vi "Obtain Thread.vi"(8 "error in (no error)":errorcluster, 9 "timeout in ms (0)":i32 format="%d ms", 11 "Thread Pool in":refnum<class "Thread Pool.lvclass">) -> (0 "error out":errorcluster, 1 "timed out?":bool, 2 "Thread":refnum<class "Thread.lvclass">, 3 "Thread Pool out":refnum<class "Thread Pool.lvclass">)   [LabVIEW 2017, in "DSF Core.lvlib" / "Thread Pool.lvclass"]
uses:
  Thread Pool.lvclass
  Thread/Thread.lvclass
  Thread Pool.lvclass/Thread Pool.ctl
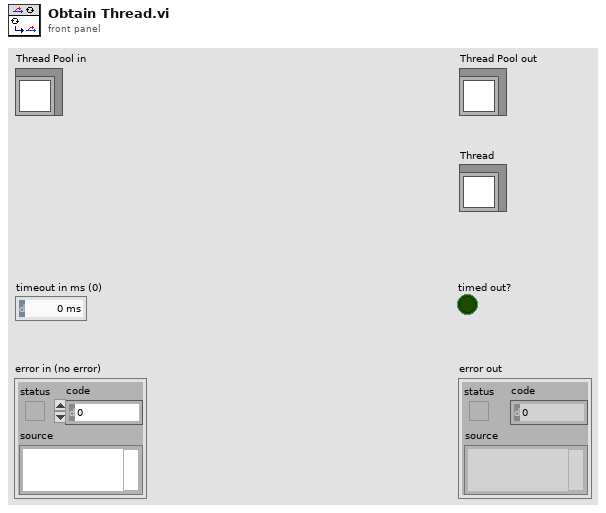
[diagram p1: front panel]
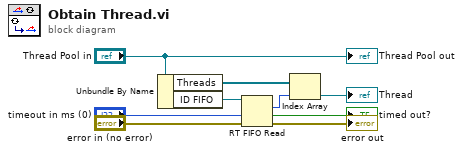
[diagram p0: block diagram]
diagram:
  n1 = Unbundle By Name("Thread Pool in") -> ("Threads"=w5:refnum<class "Thread.lvclass">[], "ID FIFO"=w8:refnum<k33>)
  n2 = RT FIFO Read(0:w8, 2:"timeout in ms (0)", 3:"error in (no error)") -> (9:w4:i32, 10:→"timed out?":bool, 11:→"error out":errorcluster)  [unwired: 1 in, 2 out]
  n3 = Index Array(array=w5, index=w4) -> (element=→"Thread":refnum<class "Thread.lvclass">)
  "Thread Pool out" <- "Thread Pool in"
